vi "Global 2.vi"() -> ()   [LabVIEW 2016]
panel:
  in  "RD Encoder Distance":dbl
  in  "LD Encoder Distance":dbl
  in  "Gyro":dbl
  in  "Shooter Velocity":dbl
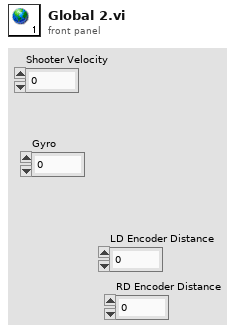
[diagram p1: front panel]
diagram:
